vi "mode_comparison_(subvi).vi"(1 "input image":path, 2 "beam cluster":T1 {"wavelength (in m)" format="%.2f"; "represented height (in m)" format="%.2f"; "represented width (in m)" format="%.2f"; "amplitude matrix" format="%.2f"}) -> (0 "Fidelity":dbl format="%#_4g")   [LabVIEW 2015]
panel:
  out "Simulation":dbl[][](graph)
  out "Image":dbl[][](graph)
  out "Difference":dbl[][](graph)
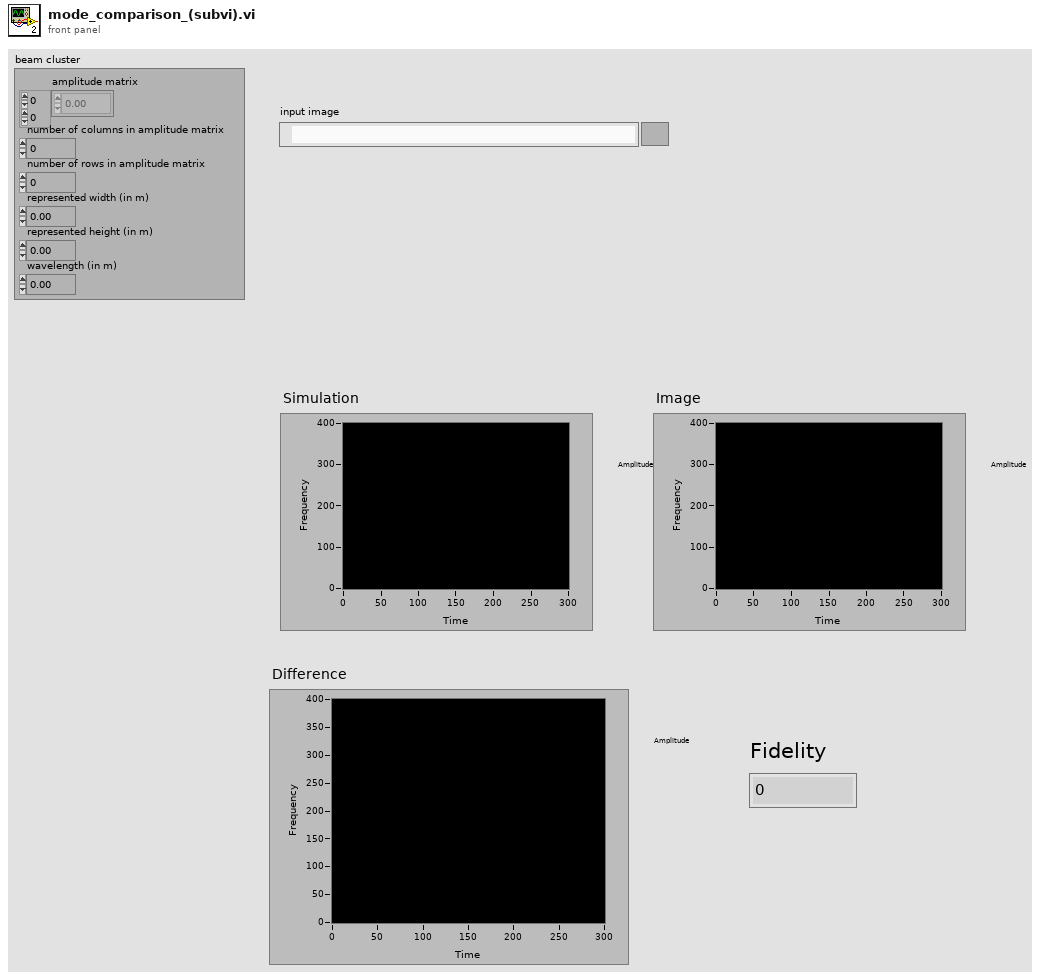
[diagram p1: front panel]
types:
  T1 = cluster{"amplitude matrix":cdb[][], "number of columns in amplitude matrix":i32, "number of rows in amplitude matrix":i32, "represented width (in m)":dbl, "represented height (in m)":dbl, "wavelength (in m)":dbl}
  T2 = typedef "imagedata.ctl" = cluster{"image type":i32, "image depth":i32, "image":u8[], "mask":u8[], "colors":u32[], "Rectangle":cluster{"left":i16, "top":i16, "right":i16, "bottom":i16}}
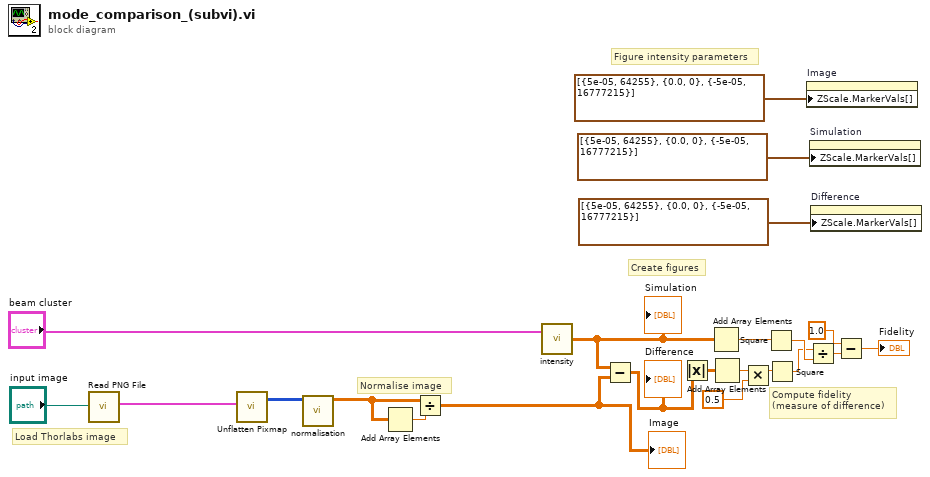
[diagram p0: block diagram]
diagram:
  # "Compute fidelity\n(measure of difference)"
  # "Create figures"
  # "Figure intensity parameters"
  # "Load Thorlabs image"
  # "Normalise image"
  n1 = call <vilib>:"Read PNG File.vi"("path to PNG file"="input image") -> ("image data"=w18:T2)  [unwired: 8 in, 2 out]
  n2 = call <vilib>:"Unflatten Pixmap.vi"("image data"=w18) -> ("24-bit pixmap"=w21:u32[][])  [unwired: 4 in, 6 out]
  n3 = call "normalisation.vi"("intensity matrix"=w21) -> ("Array"=w20:dbl[][])  [unwired: 10 in]
  n4 = Add Array Elements(numeric array=w20) -> (sum=w19:dbl)
  n5 = Divide(x=w20, y=w19) -> (x/y=w5:dbl[][])
  "Image" <- w5
  n6 = call <userlib>:"intensity.vi"("beam cluster"="beam cluster") -> ("intensity matrix"=w6:dbl[][])
  "Simulation" <- w6
  n7 = Subtract(x=w6, y=w5) -> (x-y=w7:dbl[][])
  "Difference" <- w7
  n8 = Absolute Value(x=w7) -> (abs(x)=w8:dbl[][])
  n9 = Add Array Elements(numeric array=w6) -> (sum=w14:dbl)
  n10 = Add Array Elements(numeric array=w8) -> (sum=w4:dbl)
  n11 = Multiply(x=w4, y=0.5) -> (x*y=w3:dbl)
  n12 = Square(x=w14) -> (x^2=w13:dbl)
  n13 = Square(x=w3) -> (x^2=w9:dbl)
  n14 = property on="Image" class="IntGraph (strict)"("ZScale.MarkerVals[]"=cluster{dbl, u32}[] [{5e-05, 64255}, {0.0, 0}, {-5e-05, 16777215}] ("Z Scale.Marker Values[]")) -> ()  [unwired: 2 in, 2 out]
  n15 = Divide(x=w9, y=w13) -> (x/y=w12:dbl)
  n16 = property on="Simulation" class="IntGraph (strict)"("ZScale.MarkerVals[]"=cluster{dbl, u32}[] [{5e-05, 64255}, {0.0, 0}, {-5e-05, 16777215}] ("Z Scale.Marker Values[]")) -> ()  [unwired: 2 in, 2 out]
  n17 = property on="Difference" class="IntGraph (strict)"("ZScale.MarkerVals[]"=cluster{dbl, u32}[] [{5e-05, 64255}, {0.0, 0}, {-5e-05, 16777215}] ("Z Scale.Marker Values[]")) -> ()  [unwired: 2 in, 2 out]
  n18 = Subtract(x=1.0, y=w12) -> (x-y=→"Fidelity":dbl)
